vi "GT Get Follow Virtual Seg.vi"(6 "fifo":i16, 7 "pAxis":i16, 8 "error in (no error)":errorcluster caption="错误输入（无错误）", 9 "pSegment":i16, 10 "profile":i16, 11 "cardNum":i16) -> (0 "error out":errorcluster caption="错误输出", 1 "pSegment out":i16, 3 "function return":i16, 5 "pAxis out":i16)   [LabVIEW 2020, in "gts1.lvlib"]
doc: "GT_API GT_GetFollowVirtualSeg(short cardNum,short profile,short *pSegment,short *pAxis,short fifo);"
uses:
  gts1.lvlib
  dll/32bit/multi_card/gts.dll
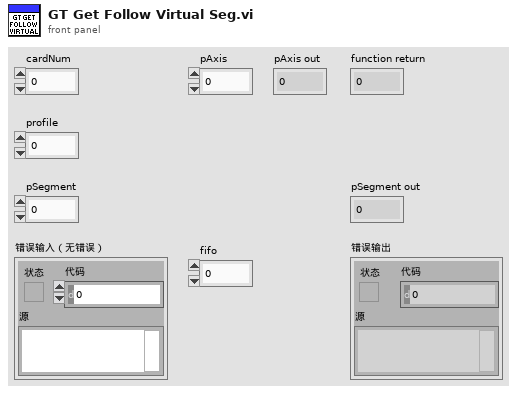
[diagram p1: front panel]
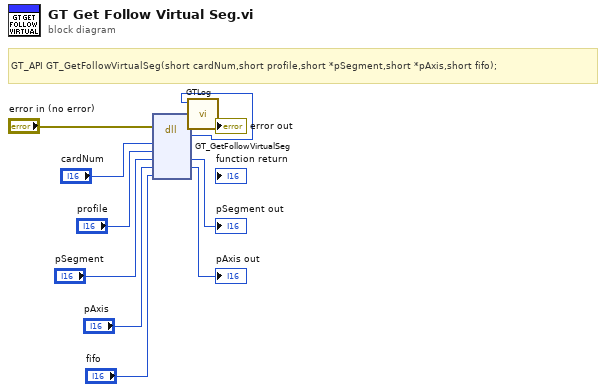
[diagram p0: block diagram]
diagram:
  # "GT_API GT_GetFollowVirtualSeg(short cardNum,short profile,short *pSegment,short *pAxis,short fifo);"
  n1 = dll-call lib="C:/1228/dll/32bit/multi_card/gts.dll" fn="GT_GetFollowVirtualSeg"(error in="error in (no error)", "cardNum"="cardNum", "profile"="profile", "pSegment"="pSegment", "pAxis"="pAxis", "fifo"="fifo") -> (error out=w3:errorcluster, w1:i16, "pSegment"=→"pSegment out":i16, "pAxis"=→"pAxis out":i16)  [unwired: 5 in, 1 out]
  n2 = call "GTLog.vi"("error in (no error)"=w3, "Numeric"=w1) -> ("error out"=→"error out":errorcluster)  [unwired: 9 in]
